vi "Renishaw-XL80_GetSerialNumber.vi"(8 "error in (no error)":errorcluster, 11 "Renishaw-XL80_EMU in":refnum<class "Renishaw-XL80_EMU.lvclass">) -> (0 "error out":errorcluster, 2 "DX10SerialNumber":string, 3 "Renishaw-XL80_EMU out":refnum<class "Renishaw-XL80_EMU.lvclass">)   [LabVIEW 2024, in "Renishaw-XL80_EMU.lvclass"]
doc: "This read only property returns the serial number of the DX10.\n\nDefinition\nHRESULTget_DX10SerialNumber( [out, retval] BSTR* pVal);\nParameters\npVal\nA variable that will be set to the serial number of the DX10. \nComments\nThis property will return an empty string if the client has not previously connected to a DX10 by calling Connect.\n\nThe property will normally return an HRESULT of S_OK. However, it will return E_POINTER if the client supplies a null pointer for pVal, and in extremely low memory conditions it will return E_NOMEMORY.\n\nSee Also"
uses:
  Renishaw-XL80_EMU.lvclass
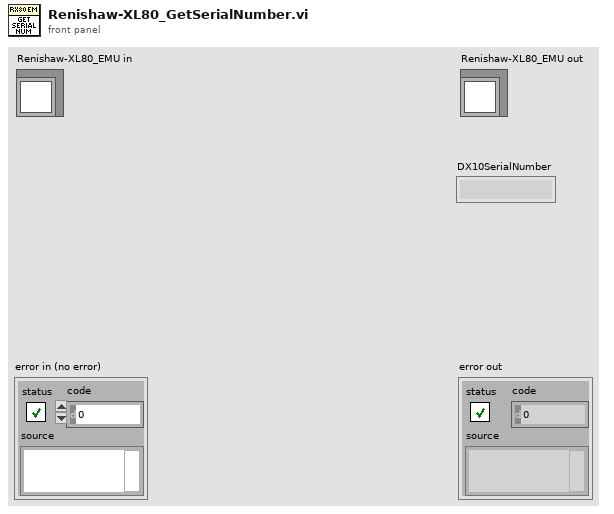
[diagram p1: front panel]
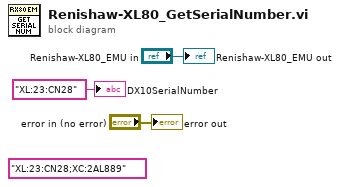
[diagram p0: block diagram]
diagram:
  (unwired) "XL:23:CN28;XC:2AL889" ("DX10SerialNumber")
  "error out" <- "error in (no error)"
  "Renishaw-XL80_EMU out" <- "Renishaw-XL80_EMU in"
  "DX10SerialNumber" <- "XL:23:CN28" ("DX10SerialNumber")
